vi "Get from queue.vi"(8 "error in (no error)":errorcluster, 10 "timeout in ms (-1)":i32=-1, 11 "Message in":refnum<class "Message.lvclass">) -> (0 "error out":errorcluster, 2 "Data":variant, 3 "Message out":refnum<class "Message.lvclass">)   [LabVIEW 2015, in "Message.lvclass"]
uses:
  Message.lvclass
  Message.lvclass/Message.ctl
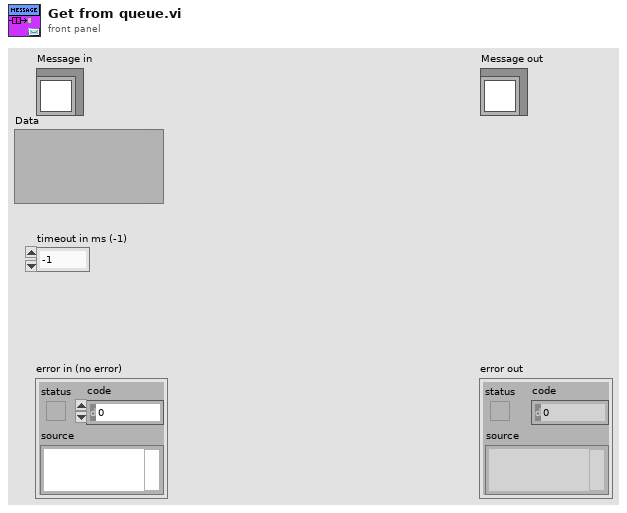
[diagram p1: front panel]
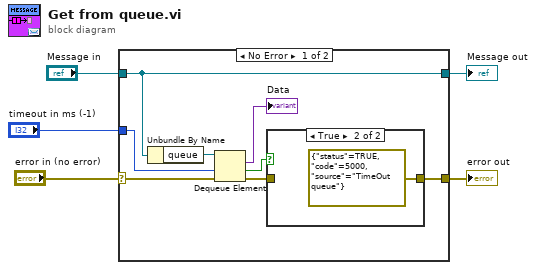
[diagram p0: block diagram]
diagram:
  n1 = case shown="No Error" "error in (no error)" {
    selector: "error in (no error)" -> [w13 w17]
    tunnel: [w9 w17] -> w4
    tunnel: [w12 w16] -> w2
    tunnel: "Message in" -> [w12 w16]
    tunnel: "timeout in ms (-1)" -> [w6 _]
    frame No Error {
      n2 = Unbundle By Name(w12) -> ("queue"=w7:refnum<queue>)
      n3 = Dequeue Element(queue=w7, timeout in ms (-1)=w6, error in (no error)=w13) -> (element=→"Data":variant, timed out?=w10:bool, error out=w8:errorcluster)  [unwired: 1 out]
      n4 = case shown="True" w10 {
        tunnel: [w14 errorcluster {"status"=TRUE, "code"=5000, "source"="TimeOut queue"} ("error out")] -> w9
        tunnel: w8 -> [w14 _]
        frame False {
        }
        frame True {
        }
      }
    }
    frame Error {
    }
  }
  "error out" <- w4
  "Message out" <- w2
